vi "Auto Reset in Change.vi"(8 "error in (no error)":errorcluster, 11 "Auto Reset":bool) -> (0 "error out":errorcluster)   [LabVIEW 2019]
uses:
  CLD 2 Time Mode.ctl
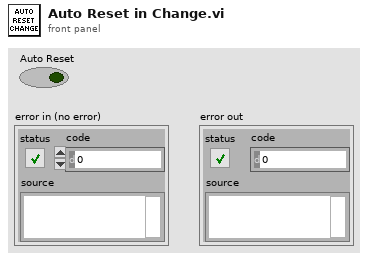
[diagram p1: front panel]
types:
  T1 = typedef "CLD 2 Time Mode.ctl" = enum16{"Reset", "Read Status", "Auto Reset and Status", "Update Target"}
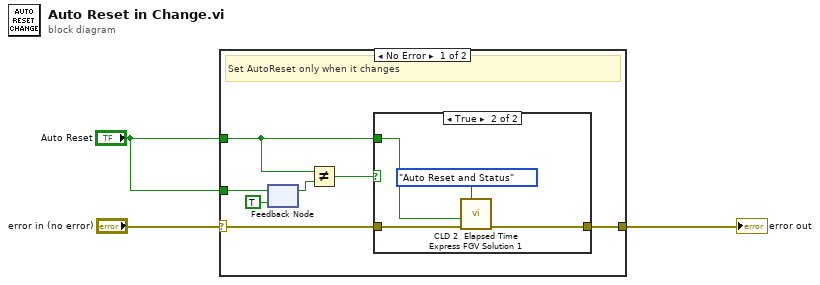
[diagram p0: block diagram]
diagram:
  n1 = case shown="No Error" "error in (no error)" {
    selector: "error in (no error)" -> [w10 w16]
    tunnel: [w9 w16] -> w2
    tunnel: "Auto Reset" -> [w8 _]
    tunnel: "Auto Reset" -> [w4 _]
    frame No Error {
      # "Set AutoReset only when it changes"
      n2 = feedback-in #1(w8) -> ()
      n3 = feedback #1(TRUE ("Auto Reset")) -> (w7:bool)
      n4 = Not Equal?(x=w4, y=w7) -> (x != y?=w5:bool)
      n5 = case shown="True" w5 {
        tunnel: w10 -> [w11 w14]
        tunnel: [w11 w13] -> w9
        tunnel: w4 -> [_ w12]
        frame False {
        }
        frame True {
          n6 = call "CLD 2  Elapsed Time Express FGV Solution 1.vi"("Timer  Mode"=CLD_2_Time_Mode."Auto Reset and Status", "error in (no error)"=w14, "Auto Reset (F)"=w12) -> ("error out"=w13:errorcluster)  [unwired: 6 in, 2 out]
        }
      }
    }
    frame Error {
    }
  }
  "error out" <- w2
